vi "Module Type.vi"(11 "Data Processor Module in":refnum<class "Data Processor Module.lvclass">) -> (2 "Module Type":string)   [LabVIEW 2020, in "VolatusData.lvlib" / "Data Processor Module.lvclass"]
uses:
  Data Processor Module.lvclass
  Data Processor Module.lvclass/Data Processor Module.ctl
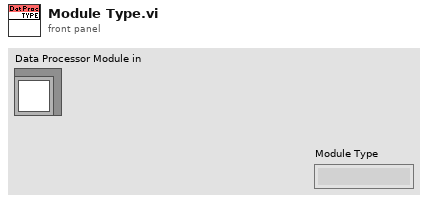
[diagram p1: front panel]
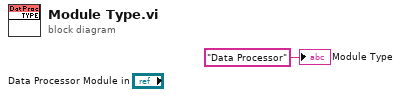
[diagram p0: block diagram]
diagram:
  "Module Type" <- "Data Processor" ("Module Type")
